vi "Write ID.vi"(8 "error in (no error)":errorcluster, 10 "ID":string, 11 "client in":refnum<class "client.lvclass">) -> (0 "error out":errorcluster, 3 "client out":refnum<class "client.lvclass">)   [LabVIEW 2016, in "client.lvlib" / "client.lvclass"]
uses:
  client.lvclass
  client.lvclass/client.ctl
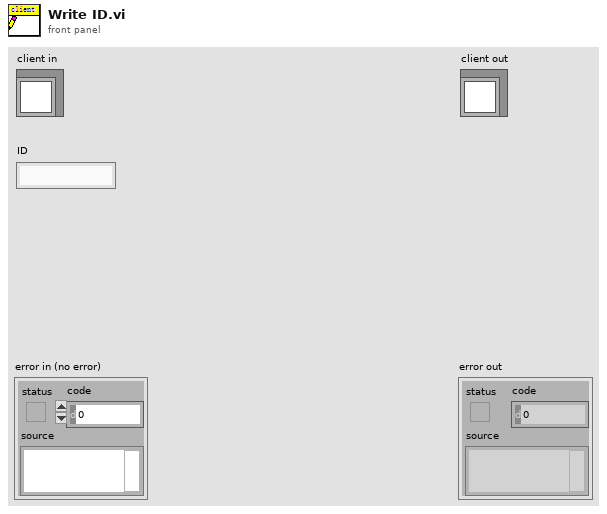
[diagram p1: front panel]
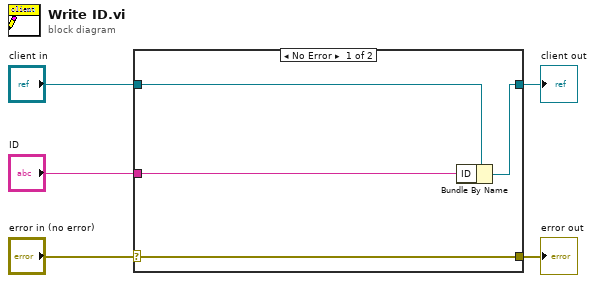
[diagram p0: block diagram]
diagram:
  n1 = case shown="No Error" "error in (no error)" {
    selector: "error in (no error)" -> [w9 w10]
    tunnel: [w9 w10] -> w4
    tunnel: [w7 w11] -> w2
    tunnel: "client in" -> [w8 w11]
    tunnel: "ID" -> [w6 _]
    frame No Error {
      n2 = Bundle By Name(cluster=w8, "ID"=w6) -> (w7:refnum<class "client.lvclass">)
    }
    frame Error {
    }
  }
  "error out" <- w4
  "client out" <- w2
